vi "OCTAL_STRING.vi"(7 "IP":string="192.168.23.100", 8 "error in (no error)":errorcluster, 9 "PARAMETERS":string, 10 "PORT":dbl=1.0 min=1.0 max=4.0 step=1.0, 11 "MASTER":dbl=1.0 min=1.0 max=10.0 step=1.0) -> (0 "error out":errorcluster, 3 "Calculated String":string caption="STRING")   [LabVIEW 2024]
uses:
  <vilib>/JDP Science/JSONtext/JSONtext.lvlib
  <userlib>/_OpenG.lib/string/string.llb/openg_string.lvlib
panel:
  in  "Multicolumn Listbox":i32(listbox)
  out "Json data":string
  # "Number to string converter"
  # "18/19/20 etc"
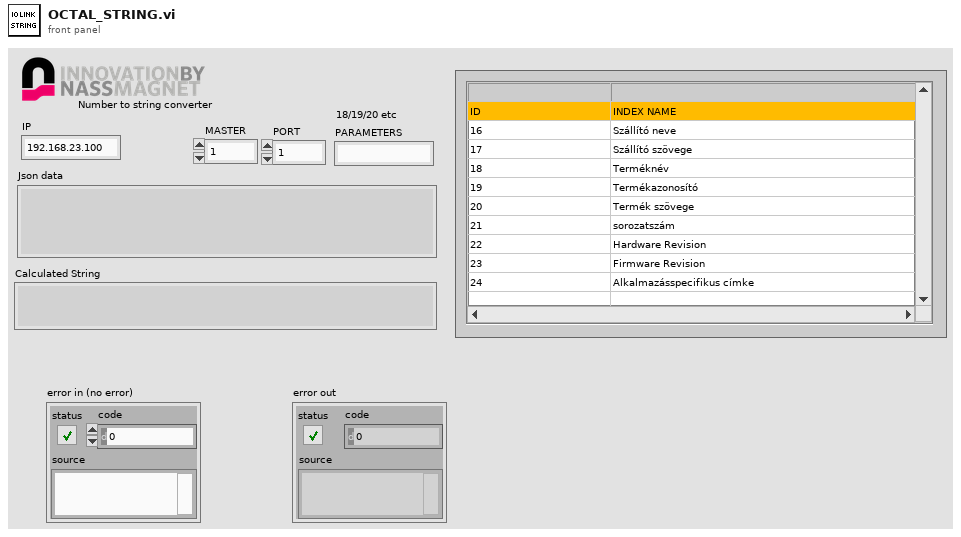
[diagram p1: front panel]
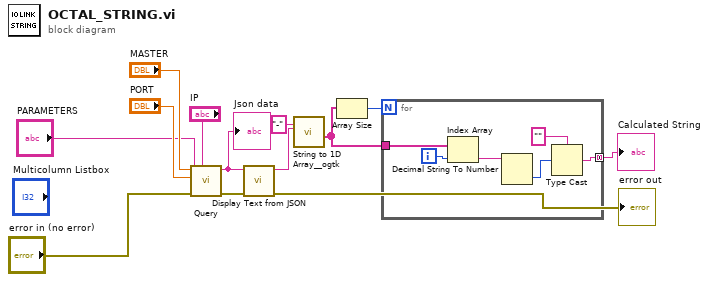
[diagram p0: block diagram]
diagram:
  n1 = call "Query.vi"("IP"="IP", "error in (no error)"="error in (no error)", "PARAMETERS"="PARAMETERS", "PORT"="PORT", "MASTER"="MASTER") -> ("error out"=w8:errorcluster, "JSON data"=w13:string)  [unwired: 5 in]
  "Json data" <- w13
  n2 = call <vilib>:"Display Text from JSON.vi"("error in (no error)"=w8, "Input JSON"=w13) -> ("error out"=→"error out":errorcluster, "Display Text"=w7:string)  [unwired: 7 in, 1 out]
  n3 = call <userlib>:"String to 1D Array__ogtk.vi"("delimiter (Tab)"="-", "string"=w7) -> ("Array of Strings"=w4:string[])  [unwired: 9 in]
  n4 = Array Size(array=w4) -> (size(s)=w3:i32)
  n5 = for {
    N: w3 -> [_]
    tunnel: w4 -> [w18]
    tunnel: [w14] -> w1 mode=concatenating
    i -> [w19]
    n6 = Index Array(array=w18, index=w19) -> (element=w17:string)
    n7 = Decimal String To Number(string=w17) -> (number=w16:i32)  [unwired: 2 in, 1 out]
    n8 = Type Cast(type="", x=w16) -> (*(type *) &x=w14:string)
  }
  "Calculated String" <- w1
